vi "Material-ConfigDialog-MessageToPageID.vi"(0 "Configuration Dialog":refnum<class "Material-ConfigDialog.lvclass">, 5 "Parameter":string, 7 "Payload":variant, 9 "PageID":string, 11 "error in":errorcluster) -> (4 "Configuration Dialog out":refnum<class "Material-ConfigDialog.lvclass">, 15 "error out":errorcluster)   [LabVIEW 2013, in "Material-ConfigDialog.lvclass"]
uses:
  Material-ConfigDialog.lvclass
  Material-ConfigDialog.lvclass/Material-ConfigDialog.ctl
  Material-ConfigDialog-Page.ctl
  Reuse Library/featherweight/Core/Messaging/Messenger.Actor/FTW-Messenger-Actor.lvclass
panel:
  # "Inputs"
  # "Outputs"
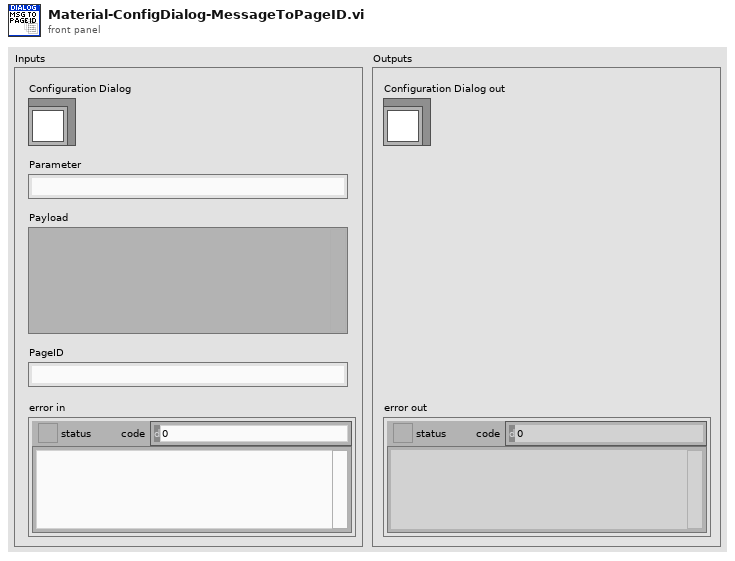
[diagram p1: front panel]
types:
  T1 = typedef "Material-ConfigDialog.lvclass/Material-ConfigDialog-Page.ctl" = cluster{"Initialized?":bool, "PageID":string, "Messenger":refnum<class "FTW-Messenger-Actor.lvclass">}
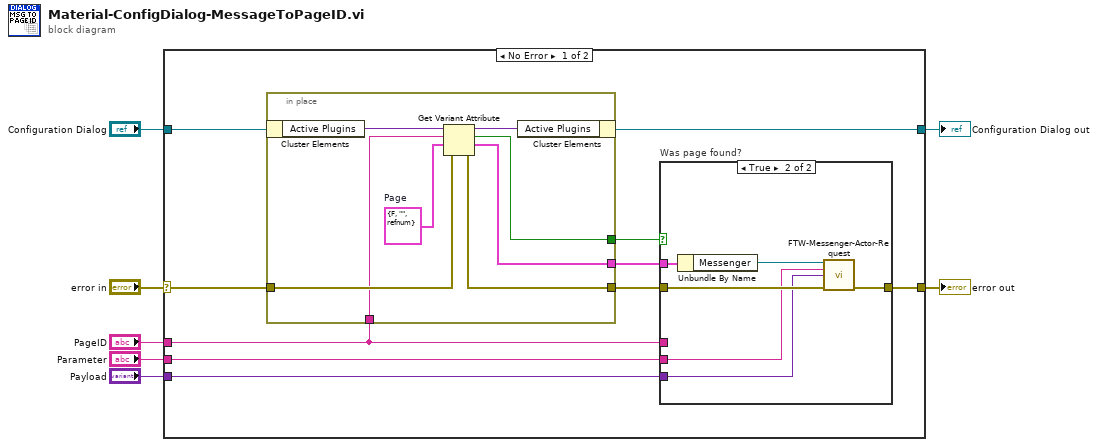
[diagram p0: block diagram]
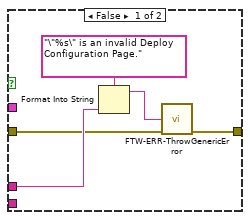
[diagram p2: hidden frame]
diagram:
  n1 = case shown="No Error" "error in" {
    selector: "error in" -> [w14 w38]
    tunnel: [w17 w38] -> w7
    tunnel: [w8 w37] -> w5
    tunnel: "Configuration Dialog" -> [w16 w37]
    tunnel: "Parameter" -> [w10 _]
    tunnel: "Payload" -> [w9 _]
    tunnel: "PageID" -> [w15 _]
    frame No Error {
      n2 = in-place {
        in-place-border: [w22] -> w13
        in-place-border: w14 -> [w23]
        in-place-border: w15 -> [w21]
        in-place-border: [w19] -> w12
        in-place-border: [w18] -> w11
        w20 = T1 {"Initialized?"=FALSE, "PageID"="", "Messenger"=refnum}  # Page
        n3 = in-place-cluster #1(w16) -> ("Active Plugins"=w25:variant)
        n4 = Get Variant Attribute(Variant=w25, name=w21, default value (empty Variant)=w20, error in=w23) -> (duplicate Variant=w24:variant, found=w19:bool, value=w18:T1, error out=w22:errorcluster)
        n5 = in-place-cluster #1("Active Plugins"=w24) -> (w8:refnum<class "Material-ConfigDialog.lvclass">)
      }
      n6 = case "Was page found?" shown="True" w12 {
        tunnel: [w27 w35] -> w17
        tunnel: w13 -> [w28 w34]
        tunnel: w15 -> [w29 _]
        tunnel: w11 -> [_ w36]
        tunnel: w10 -> [_ w32]
        tunnel: w9 -> [_ w31]
        frame False {
          n7 = Format Into String(format string="\"%s\" is an invalid Deploy Configuration Page.", w29) -> (resulting string=w26:string)  [unwired: 2 in, 1 out]
          n8 = call "FTW-ERR-ThrowGenericError.vi"("Error Message"=w26, "error in"=w28) -> ("error out"=w27:errorcluster)  [unwired: 13 in]
        }
        frame True {
          n9 = Unbundle By Name(w36) -> ("Messenger"=w33:refnum<class "FTW-Messenger-Actor.lvclass">)
          n10 = call-dynamic "FTW-Messenger-Actor-Request.vi"("Messenger"=w33, "Parameter"=w32, "Payload"=w31, "error in"=w34) -> ("error out"=w35:errorcluster)  [unwired: 10 in, 1 out]
        }
      }
    }
    frame Error {
    }
  }
  "error out" <- w7
  "Configuration Dialog out" <- w5
